vi "BK Precision 913XX Triggered Output.vi"() -> ()   [LabVIEW 2012]
doc: "This example shows how to configure trigger and capture pre-trigger and post-trigger output measurements."
uses:
  <instrlib>/BK Precision 913XX/BK Precision 913XX.lvlib
panel:
  out "Post-trigger Power Level (W)":dbl format="%.4g"
  out "Post-trigger Voltage Level (V)":dbl format="%.4g"
  out "Post-trigger Current Level (A)":dbl format="%.4g"
  out "Pre-trigger Power Level (W)":dbl format="%.4g"
  out "Pre-trigger Voltage Level (V)":dbl format="%.4g"
  out "Pre-trigger Current Level (A)":dbl format="%.4g"
  in  "Triggered Current Limit (0.0 A)":dbl min=0.0 max=25.0 step=1.0 format="%.3f"
  in  "Triggered Voltage Level (0.000 V)":dbl min=0.0 max=61.0 step=0.001 format="%.3f"
  in  "Channel (1:1)":u16(ring)=1 items=["1"=1, "2"=2, "3"=3]
  in  "Current Limit (0.0 A)":dbl min=0.0 max=25.0 step=1.0 format="%.3f"
  in  "Voltage Level (0.0 V)":dbl format="%.3g"
  in  "VISA resource name":refnum<visa-resource-name>
  # "(c) 2015 B&K Precision Corporation.  ALL RIGHTS RESERVED."
  # "Initial Voltage Settings"
  # "Triggered Settings"
  # "Post-trigger Levels"
  # "Pre-trigger Levels"
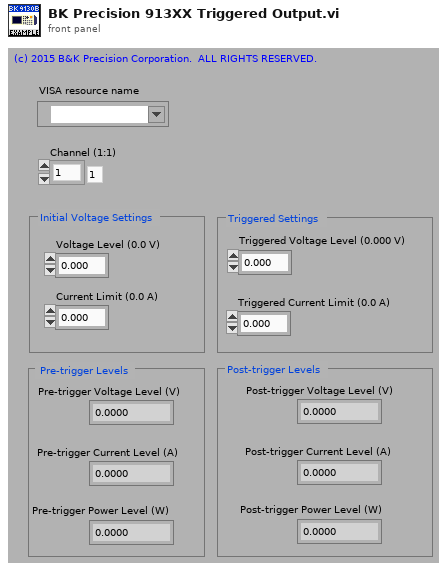
[diagram p1: front panel]
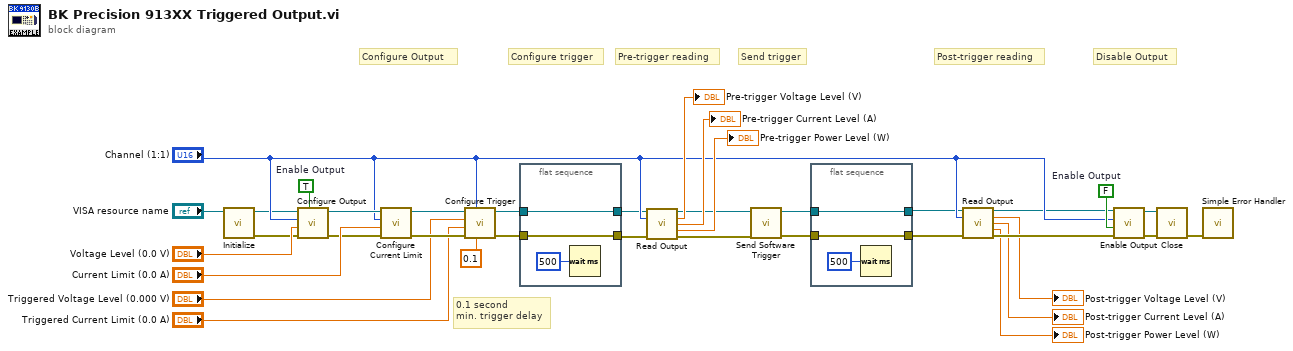
[diagram p0: block diagram]
diagram:
  w27 = FALSE  # Enable Output
  w32 = TRUE  # Enable Output
  # "Send trigger"
  # "Configure trigger"
  # "Post-trigger reading"
  # "0.1 second \nmin. trigger delay"
  # "Disable Output"
  # "Pre-trigger reading"
  # "Configure Output"
  n1 = call <instrlib>:"Initialize.vi"("VISA resource name"="VISA resource name") -> ("error out"=w10:errorcluster, "VISA resource name out"=w9:refnum<visa-resource-name>)  [unwired: 9 in]
  n2 = call <instrlib>:"Configure Output.vi"("Enable Channel Output (F: False)"=w32, "error in (no error)"=w10, "Voltage Level (0.0 V)"="Voltage Level (0.0 V)", "Channel (1:1)"="Channel (1:1)", "VISA resource name"=w9) -> ("error out"=w28:errorcluster, "VISA resource name out"=w29:refnum<visa-resource-name>)  [unwired: 5 in]
  n3 = call <instrlib>:"Configure Current Limit.vi"("error in (no error)"=w28, "Current Limit (0.0 A)"="Current Limit (0.0 A)", "Channel (1:1)"="Channel (1:1)", "VISA resource name"=w29) -> ("error out"=w25:errorcluster, "VISA resource name out"=w26:refnum<visa-resource-name>)  [unwired: 6 in]
  n4 = call <instrlib>:"Configure Trigger.vi"("Trigger Delay (0.1 s)"=0.1, "Channel (1:1)"="Channel (1:1)", "error in (no error)"=w25, "Triggered Current Limit (0.0 A)"="Triggered Current Limit (0.0 A)", "Triggered Voltage Level (0.000 V)"="Triggered Voltage Level (0.000 V)", "VISA resource name"=w26) -> ("error out"=w7:errorcluster, "VISA resource name out"=w6:refnum<visa-resource-name>)  [unwired: 4 in]
  n5 = flat-sequence {
    tunnel: [w38] -> w8
    tunnel: w7 -> [w38]
    tunnel: w6 -> [w37]
    tunnel: [w37] -> w5
    frame #0 {
      n6 = Wait (ms)(milliseconds to wait=u32 500) -> ()  [unwired: 1 out]
    }
  }
  n7 = call <instrlib>:"Read Output.vi"("VISA resource name"=w5, "Channel (1:Channel 1)"="Channel (1:1)", "error in (no error)"=w8) -> ("VISA resource name out"=w18:refnum<visa-resource-name>, "Actual Voltage Level (V)"=→"Pre-trigger Voltage Level (V)":dbl, "Actual Current Level (A)"=→"Pre-trigger Current Level (A)":dbl, "Actual Power Level (W)"=→"Pre-trigger Power Level (W)":dbl, "error out"=w17:errorcluster)  [unwired: 8 in]
  n8 = call <instrlib>:"Send Software Trigger.vi"("error in (no error)"=w17, "VISA resource name"=w18) -> ("error out"=w3:errorcluster, "VISA resource name out"=w4:refnum<visa-resource-name>)  [unwired: 8 in]
  n9 = flat-sequence {
    tunnel: [w41] -> w2
    tunnel: w3 -> [w41]
    tunnel: w4 -> [w40]
    tunnel: [w40] -> w1
    frame #0 {
      n10 = Wait (ms)(milliseconds to wait=u32 500) -> ()  [unwired: 1 out]
    }
  }
  n11 = call <instrlib>:"Read Output.vi"("VISA resource name"=w1, "Channel (1:Channel 1)"="Channel (1:1)", "error in (no error)"=w2) -> ("VISA resource name out"=w15:refnum<visa-resource-name>, "Actual Voltage Level (V)"=→"Post-trigger Voltage Level (V)":dbl, "Actual Current Level (A)"=→"Post-trigger Current Level (A)":dbl, "Actual Power Level (W)"=→"Post-trigger Power Level (W)":dbl, "error out"=w14:errorcluster)  [unwired: 8 in]
  n12 = call <instrlib>:"Enable Output.vi"("error in (no error)"=w14, "Enable Output (F: False)"=w27, "Channel (1:1)"="Channel (1:1)", "VISA resource name"=w15) -> ("error out"=w33:errorcluster, "VISA resource name out"=w34:refnum<visa-resource-name>)  [unwired: 6 in]
  n13 = call <instrlib>:"Close.vi"("error in (no error)"=w33, "VISA resource name"=w34) -> ("error out"=w35:errorcluster)  [unwired: 9 in]
  n14 = call <vilib>:"Simple Error Handler.vi"("error in (no error)"=w35) -> ()  [unwired: 4 in, 5 out]
